vi "Python_SaveFile.vi"(8 "File text":string, 9 "File name":string, 10 "Python version":string="3.9", 11 "Port":string) -> (2 "Console":string)   [LabVIEW 2020]
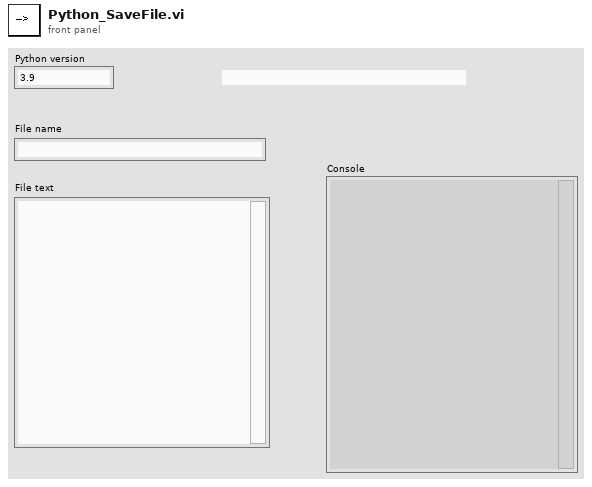
[diagram p1: front panel]
types:
  T1 = typedef "PythonCtrl.ctl" = cluster{"session":refnum<k35>, "PyPath":path}
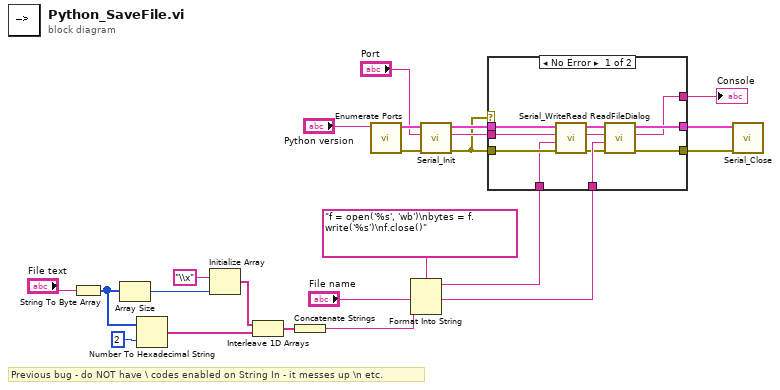
[diagram p0: block diagram]
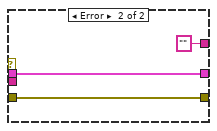
[diagram p2: hidden frame]
diagram:
  # "Previous bug - do NOT have \\ codes enabled on String In - it messes up \\n etc."
  n1 = String To Byte Array(string="File text") -> (unsigned byte array=w13:u8[])
  n2 = Array Size(array=w13) -> (size(s)=w12:i32)
  n3 = Number To Hexadecimal String(1:i16 2 ("width (-)"), 2:w13) -> (0:w14:string[])
  n4 = Initialize Array("\\x", w12) -> (w10:string[])
  n5 = Interleave 1D Arrays(w10, w14) -> (w9:string[])
  n6 = Concatenate Strings(w9) -> (w7:string)
  n7 = call "Enumerate Ports.vi"("Python version"="Python version") -> ("error out"=w20:errorcluster, "Python"=w22:T1)  [unwired: 7 in, 2 out]
  n8 = Format Into String(format string="f = open('%s', 'wb')\nbytes = f.write('%s')\nf.close()" ("function name"), "File name", w7) -> (resulting string=w5:string)  [unwired: 2 in, 1 out]
  n9 = call "Serial_Init.vi"("error in (no error)"=w20, "Port"="Port", "Python"=w22) -> ("error out"=w1:errorcluster, "Console"=w17:string, "Python out"=w18:T1)  [unwired: 6 in]
  n10 = case shown="No Error" w1 {
    tunnel: w18 -> [w32 w35]
    tunnel: w1 -> [w31 w34]
    tunnel: w17 -> [w30 _]
    tunnel: "File name" -> [w29 _]
    tunnel: w5 -> [w28 _]
    tunnel: [w25 w34] -> w4
    tunnel: [w24 w35] -> w3
    tunnel: [w23 "" ("Console")] -> w2
    frame No Error {
      n11 = call "Serial_WriteRead.vi"("error in (no error)"=w31, "Code"=w28, "Console In"=w30, "Python"=w32) -> ("error out"=w27:errorcluster, "Console"=w26:string, "Python"=w24:T1)  [unwired: 5 in]
      n12 = call "ReadFileDialog.vi"("error in (no error)"=w27, "File name"=w29, "Console in"=w26, "Python in"=w24) -> ("error out"=w25:errorcluster, "Console"=w23:string)  [unwired: 6 in]
    }
    frame Error {
    }
  }
  "Console" <- w2
  n13 = call "Serial_Close.vi"("error in (no error)"=w4, "Python in"=w3) -> ()  [unwired: 10 in]
